vi "Target Lookup Setpoint.vi"(11 "Phase":dbl) -> (3 "Setpoint":dbl)   [LabVIEW 2018]
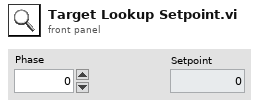
[diagram p1: front panel]
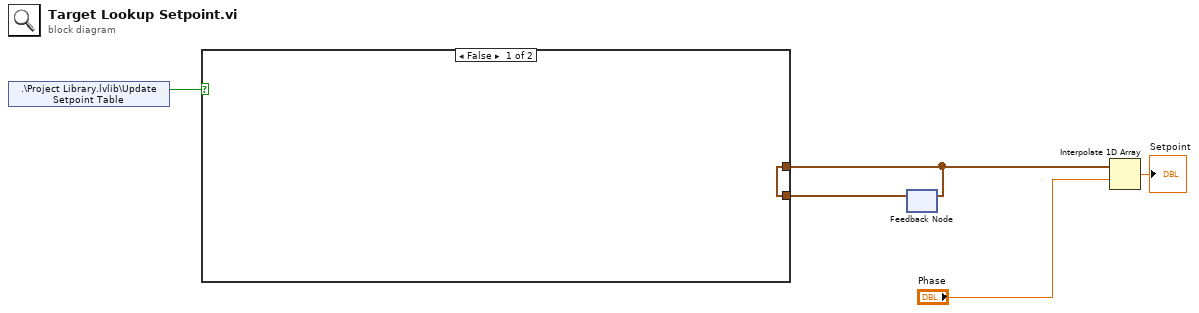
[diagram p0: block diagram]
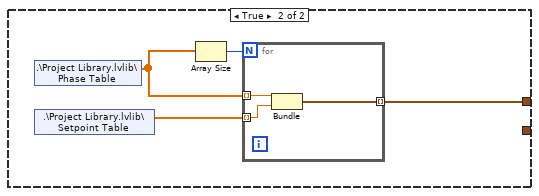
[diagram p2: hidden frame]
diagram:
  n1 = shared-variable ".\\Project Library.lvlib\\Update Setpoint Table"() -> (w3:bool)  [unwired: 1 in, 1 out]
  n2 = feedback #1() -> (w2:cluster{"Numeric":dbl, "Numeric":dbl}[])  [unwired: 1 in]
  n3 = case shown="False" w3 {
    tunnel: [w6 w7] -> w1
    tunnel: w2 -> [w6 _]
    frame False {
    }
    frame True {
      n4 = shared-variable ".\\Project Library.lvlib\\Phase Table"() -> (w9:dbl[])  [unwired: 1 in, 1 out]
      n5 = shared-variable ".\\Project Library.lvlib\\Setpoint Table"() -> (w8:dbl[])  [unwired: 1 in, 1 out]
      n6 = Array Size(array=w9) -> (size(s)=w10:i32)
      n7 = for {
        N: w10 -> [_]
        tunnel: w9 -> [w13] mode=indexing
        tunnel: w8 -> [w12] mode=indexing
        tunnel: [w11] -> w7 mode=indexing
        n8 = Bundle("Numeric"=w13, "Numeric"=w12) -> (w11:cluster{"Numeric":dbl, "Numeric":dbl})  [unwired: 1 in]
      }
    }
  }
  n9 = feedback-in #1(w1) -> ()
  n10 = Interpolate 1D Array(1:"Phase", 2:w1) -> (0:→"Setpoint":dbl)
